vi "DisConnect.vi"(4 "error in (no error)":errorcluster, 7 ".NET Reference in":refnum<k24>) -> (0 "error out":errorcluster, 3 "Reference out":refnum<k24>)   [LabVIEW 2017]
uses:
  LV_IL_Sample/DLL/InstrumentDLL.dll
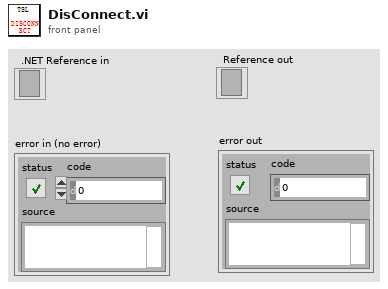
[diagram p1: front panel]
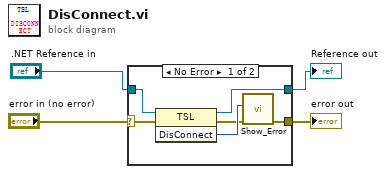
[diagram p0: block diagram]
diagram:
  n1 = case shown="No Error" "error in (no error)" {
    selector: "error in (no error)" -> [w5 w12]
    tunnel: [w6 w12] -> w4
    tunnel: [w10 w11] -> w3
    tunnel: ".NET Reference in" -> [w9 w11]
    frame No Error {
      n2 = invoke on="调用节点" class="TSL" method="DisConnect"(reference=w9, error in=w5) -> (reference out=w10:refnum<k24>, error out=w7:errorcluster, "DisConnect"=w8:i32)  [unwired: 1 in]
      n3 = call "Show_Error.vi"("error in (no error)"=w7, "Error"=w8) -> ("error out"=w6:errorcluster)  [unwired: 9 in]
    }
    frame Error {
    }
  }
  "Reference out" <- w3
  "error out" <- w4
